vi "Thermal_Cycler_v0.3.vi"() -> ()   [LabVIEW 2023]
uses:
  <vilib>/Instr/_visa.llb/VISA Configure Serial Port (Instr).vi
panel:
  out "Flat Cycle Count":dbl
  out "Cold Count Readout":i32
  in  "Cold Count":i32
  in  "Cold Count Trigger":i32
  in  "Hot Count":i32
  in  "Hot Count Trigger":i32
  out "Full Temp Graph":dbl(graph)
  out "Cycle Temp Graph":dbl(graph)
  out "Current Cycle":i32
  out "Cycle Name":string
  out "Cooling":bool
  out "Heating":bool
  out "DONE":bool
  out "Soak High Adjusted":string
  out "Soak Low Adjusted":string
  in  "Multiplier":i32=60000
  out "Cycle Time in Minutes Adjusted":i32
  out "Temp Readout":dbl
  out "test read":string
  out "CYCLING":bool
  out "Was temp set correctly?":string
  in  "Comms delay":i32=1500
  in  "Number of Cycles to Complete":i32=2
  in  "Cycle Time in Minutes":i32=1
  in  "Soak Low":string="40"
  in  "Soak High":string="45"
  in  "baud rate":i32=19200
  out "ON/OFF":bool
  out "?":errorcluster
  in  "COM Port":refnum<visa-resource-name>="COM3"
  # "Debugging"
  # "Serial Port and Save Data Settings"
  # "Cycle and Temperature Settings"
  # "Readouts"
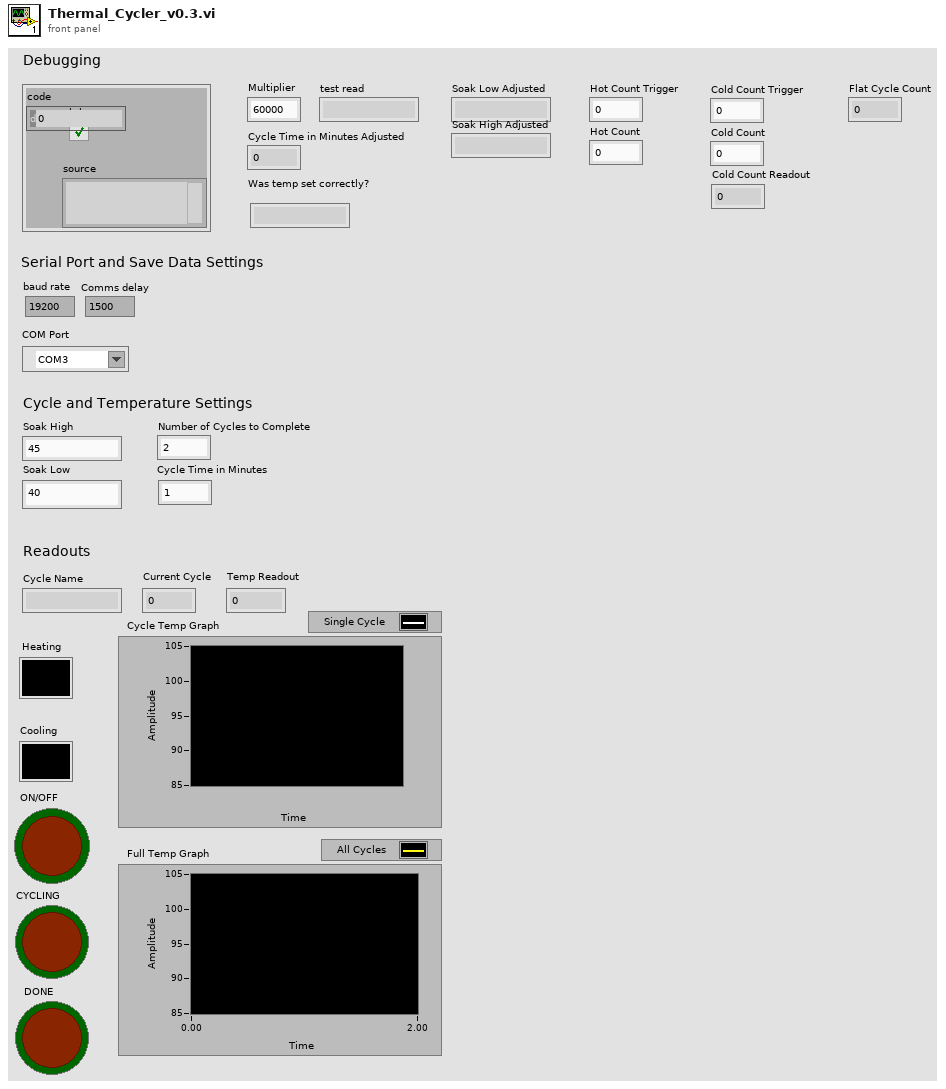
[diagram p1: front panel]
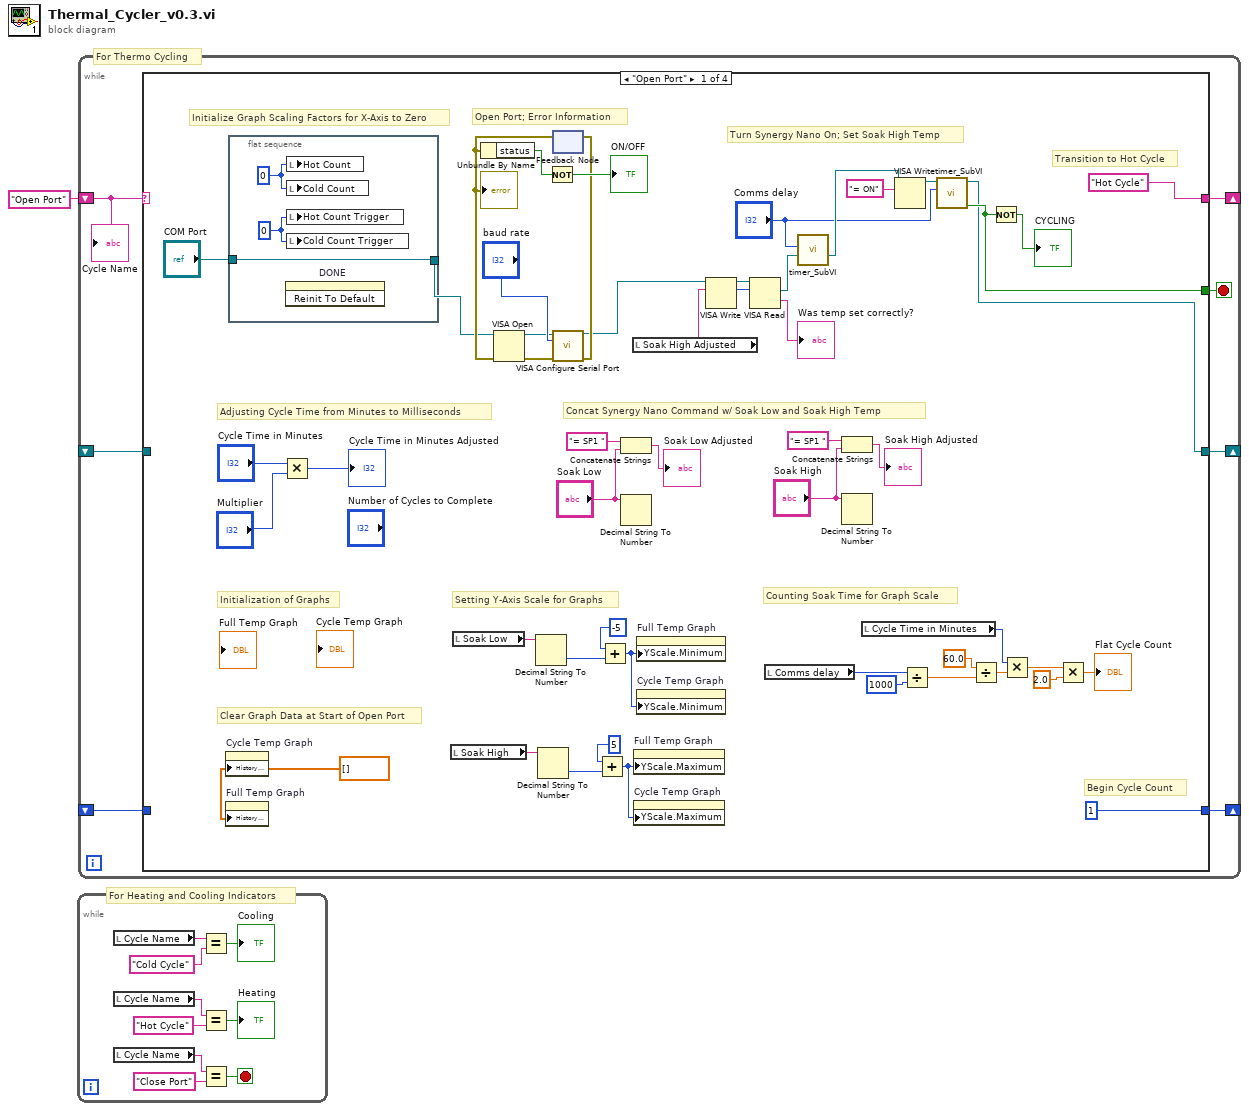
[diagram p0: block diagram]
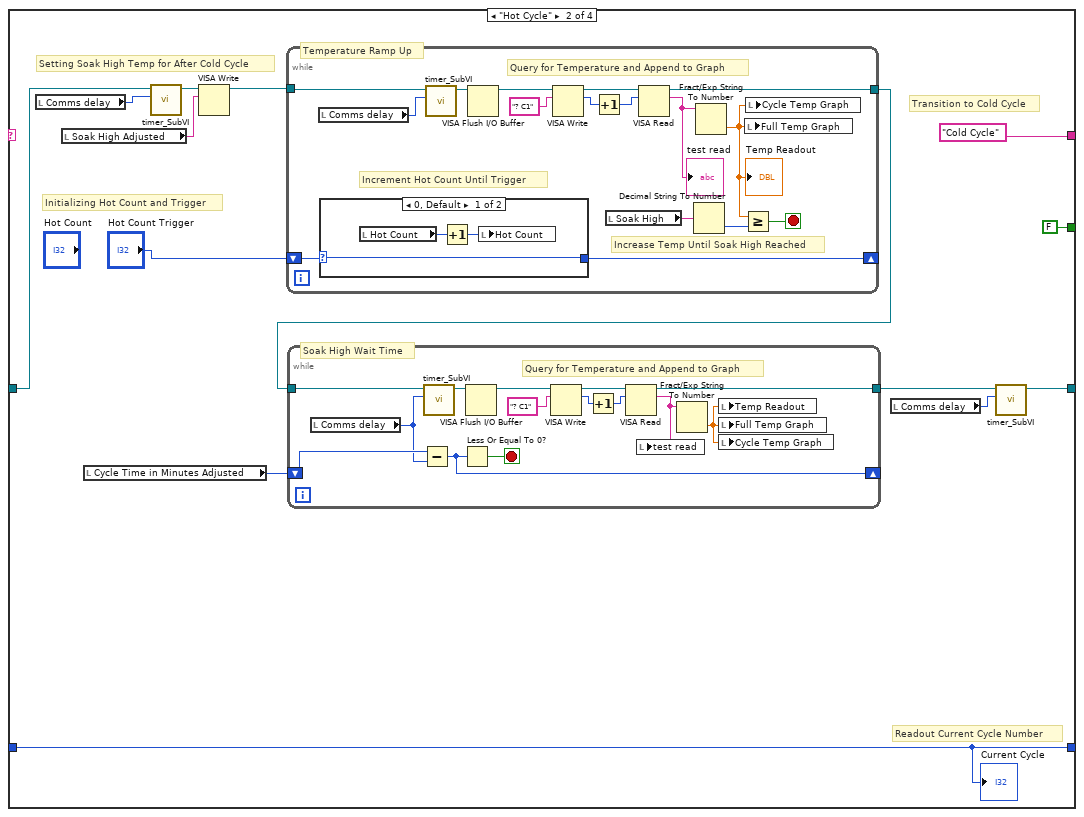
[diagram p2: hidden frame]
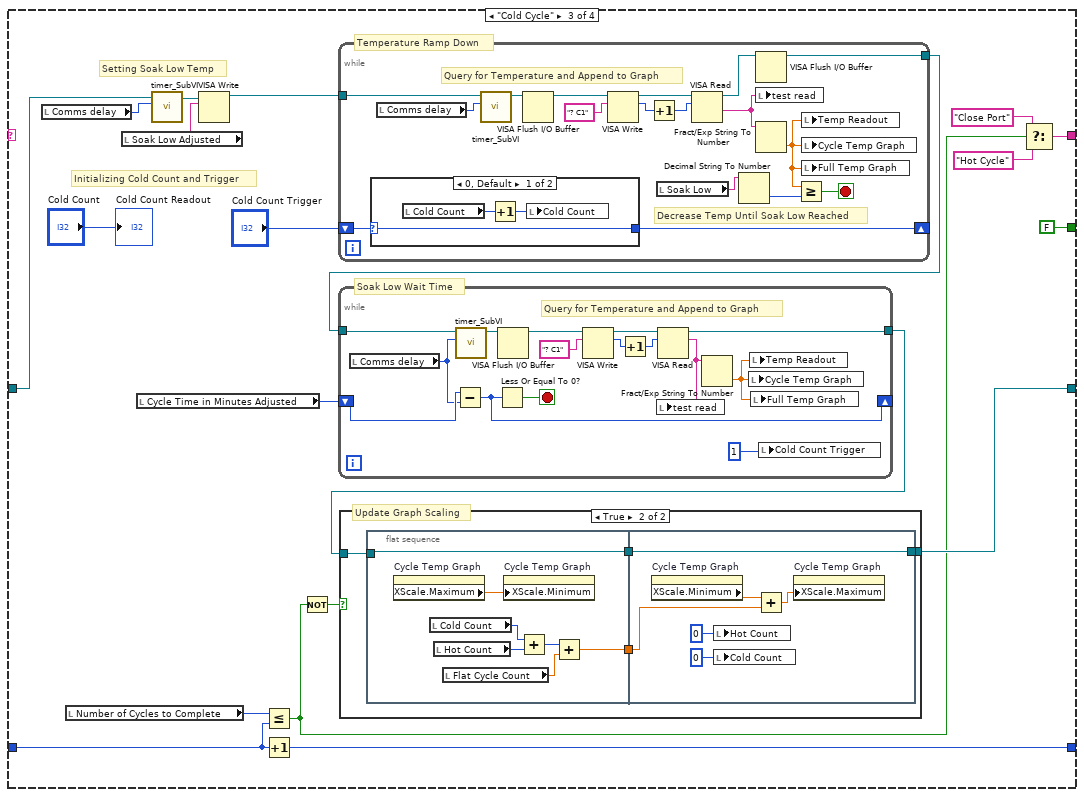
[diagram p4: hidden frame]
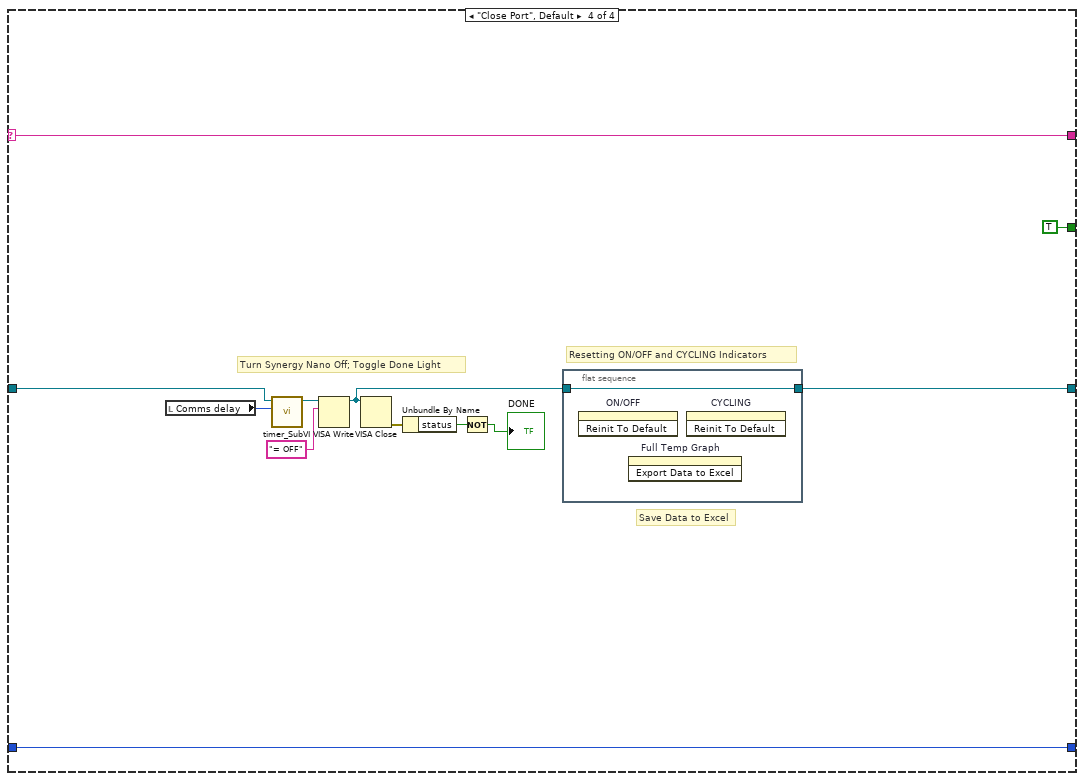
[diagram p7: hidden frame]
diagram:
  # "For Thermo Cycling"
  # "For Heating and Cooling Indicators"
  n1 = while {
    stop <- w2 stop-if-true
    n2 = local read "Cycle Name"() -> (w7:string)
    n3 = local read "Cycle Name"() -> (w10:string)
    n4 = local read "Cycle Name"() -> (w4:string)
    n5 = Equal?(x=w7, y="Cold Cycle") -> (x = y?=→"Cooling":bool)
    n6 = Equal?(x=w10, y="Hot Cycle") -> (x = y?=→"Heating":bool)
    n7 = Equal?(x=w4, y="Close Port") -> (x = y?=w2:bool)
  }
  n8 = while {
    shift-right: [w16] -> _
    shift-left: "Open Port" -> [w11]
    shift-right: [w15] -> _
    shift-left: _ -> [w14]
    shift-right: [w13] -> _
    shift-left: _ -> [w12]
    stop <- w17 stop-if-true
    n9 = case shown="\"Open Port\"" w11 {
      selector: w11 -> [_ _ _ w205]
      tunnel: [w46 FALSE FALSE TRUE] -> w17
      tunnel: ["Hot Cycle" "Cold Cycle" w128 w205] -> w16
      tunnel: [w44 w79 w122 w194] -> w15
      tunnel: w14 -> [_ w76 w134 w202]
      tunnel: [1 ("Numeric") w73 w126 w196] -> w13
      tunnel: w12 -> [_ w73 w127 w196]
      frame "Open Port" {
        w32 = dbl[] [] ("History Data")
        # "Transition to Hot Cycle"
        # "Begin Cycle Count"
        # "Turn Synergy Nano On; Set Soak High Temp"
        # "Open Port; Error Information"
        # "Initialize Graph Scaling Factors for X-Axis to Zero"
        # "Counting Soak Time for Graph Scale"
        # "Initialization of Graphs"
        # "Setting Y-Axis Scale for Graphs"
        # "Clear Graph Data at Start of Open Port"
        # "Adjusting Cycle Time from Minutes to Milliseconds"
        # "Concat Synergy Nano Command w/ Soak Low and Soak High Temp"
        n10 = property on="Cycle Temp Graph" class="WFChart (strict)"("History Data"=w32) -> ()  [unwired: 2 in, 2 out]
        n11 = property on="Full Temp Graph" class="WFChart (strict)"("History Data"=w32) -> ()  [unwired: 2 in, 2 out]
        n12 = flat-sequence {
          tunnel: "COM Port" -> [w71]
          tunnel: [w71] -> w30
          frame #0 {
            w69 = 0 ("Cold Count Trigger")
            w70 = 0 ("Cold Count")
            n13 = invoke on="DONE" class="Bool (strict)" method="Reinit To Default"() -> ()  [unwired: 3 in, 3 out]
            n14 = local write "Hot Count"(w70) -> ()
            n15 = local write "Cold Count"(w70) -> ()
            n16 = local write "Hot Count Trigger"(w69) -> ()
            n17 = local write "Cold Count Trigger"(w69) -> ()
          }
        }
        n18 = Multiply(x="Cycle Time in Minutes", y="Multiplier") -> (x*y=→"Cycle Time in Minutes Adjusted":i32)
        n19 = local read "Soak High"() -> (w34:string)
        n20 = local read "Soak Low"() -> (w33:string)
        n21 = Decimal String To Number(string=w33) -> (number=w41:i32)  [unwired: 2 in, 1 out]
        n22 = Decimal String To Number(string=w34) -> (number=w38:i32)  [unwired: 2 in, 1 out]
        n23 = feedback #1() -> (w60:errorcluster)  [unwired: 1 in]
        "?" <- w60
        n24 = Unbundle By Name(w60) -> ("status"=w65:bool)
        n25 = VISA Open(error in (no error)=w60, VISA resource name=w30) -> (VISA resource name=w66:refnum<visa-resource-name>, error out=w68:errorcluster)  [unwired: 3 in]
        n26 = Not(x=w65) -> (.not. x?=→"ON/OFF":bool)
        n27 = call-poly "VISA Configure Serial Port"("VISA resource name"=w66, "baud rate (9600)"="baud rate", "error in (no error)"=w68) -> ("VISA resource name out"=w47:refnum<visa-resource-name>, "error out"=w61:errorcluster)  [unwired: 11 in]
        n28 = feedback-in #1(w61) -> ()
        n29 = Add(x=5, y=w38) -> (x+y=w35:i32)
        n30 = Add(x=-5, y=w41) -> (x+y=w39:i32)
        n31 = Concatenate Strings("= SP1 ", "Soak Low") -> (→"Soak Low Adjusted":string)
        n32 = Decimal String To Number(string="Soak Low") -> ()  [unwired: 2 in, 2 out]
        n33 = local read "Soak High Adjusted"() -> (w20:string)
        n34 = property on="Full Temp Graph" class="WFChart (strict)"("YScale.Maximum"=w35) -> ()  [unwired: 2 in, 2 out]
        n35 = property on="Cycle Temp Graph" class="WFChart (strict)"("YScale.Maximum"=w35) -> ()  [unwired: 2 in, 2 out]
        n36 = property on="Full Temp Graph" class="WFChart (strict)"("YScale.Minimum"=w39) -> ()  [unwired: 2 in, 2 out]
        n37 = property on="Cycle Temp Graph" class="WFChart (strict)"("YScale.Minimum"=w39) -> ()  [unwired: 2 in, 2 out]
        n38 = VISA Write(VISA resource name=w47, write buffer=w20) -> (VISA resource name out=w48:refnum<visa-resource-name>, return count=w49:u32)  [unwired: 1 in, 1 out]
        n39 = VISA Read(VISA resource name=w48, byte count=w49) -> (VISA resource name out=w59:refnum<visa-resource-name>, read buffer=→"Was temp set correctly?":string)  [unwired: 1 in, 2 out]
        n40 = local read "Comms delay"() -> (w28:i32)
        n41 = call "timer_SubVI.vi"("Comms Delay In"="Comms delay", "VISA  in"=w59) -> ("VISA out"=w56:refnum<visa-resource-name>)  [unwired: 7 in, 2 out]
        n42 = Concatenate Strings("= SP1 ", "Soak High") -> (→"Soak High Adjusted":string)
        n43 = Decimal String To Number(string="Soak High") -> ()  [unwired: 2 in, 2 out]
        n44 = local read "Cycle Time in Minutes"() -> (w29:i32)
        n45 = VISA Write(VISA resource name=w56, write buffer="= ON") -> (VISA resource name out=w55:refnum<visa-resource-name>)  [unwired: 1 in, 2 out]
        n46 = Divide(x=w28, y=1000) -> (x/y=w25:dbl)
        n47 = call "timer_SubVI.vi"("Comms Delay In"="Comms delay", "VISA  in"=w55) -> ("bool out"=w46:bool, "VISA out"=w44:refnum<visa-resource-name>)  [unwired: 7 in, 1 out]
        n48 = Divide(x=60.0 ("y"), y=w25) -> (x/y=w24:dbl)
        n49 = Not(x=w46) -> (.not. x?=→"CYCLING":bool)
        n50 = Multiply(x=w29, y=w24) -> (x*y=w23:dbl)
        n51 = Multiply(x=w23, y=2.0) -> (x*y=→"Flat Cycle Count":dbl)
      }
      frame "Hot Cycle" {
        # "Transition to Cold Cycle"
        # "Readout Current Cycle Number"
        # "Soak High Wait Time"
        # "Initializing Hot Count and Trigger"
        # "Setting Soak High Temp for After Cold Cycle"
        # "Temperature Ramp Up"
        n52 = local read "Comms delay"() -> (w74:i32)
        n53 = local read "Soak High Adjusted"() -> (w83:string)
        n54 = local read "Cycle Time in Minutes Adjusted"() -> (w81:i32)
        n55 = call "timer_SubVI.vi"("Comms Delay In"=w74, "VISA  in"=w76) -> ("VISA out"=w75:refnum<visa-resource-name>)  [unwired: 7 in, 2 out]
        n56 = VISA Write(VISA resource name=w75, write buffer=w83) -> (VISA resource name out=w84:refnum<visa-resource-name>)  [unwired: 1 in, 2 out]
        n57 = while {
          tunnel: [w109] -> w82
          tunnel: w84 -> [w108]
          shift-right: [w100] -> _
          shift-left: "Hot Count Trigger" -> [w101]
          stop <- w112 stop-if-true
          # "Increase Temp Until Soak High Reached"
          # "Query for Temperature and Append to Graph"
          # "Increment Hot Count Until Trigger"
          n58 = local read "Comms delay"() -> (w107:i32)
          n59 = case shown="0, Default" w101 {
            selector: w101 -> [w116 w119]
            tunnel: [w116 w119] -> w100
            frame 0, Default {
              n60 = local read "Hot Count"() -> (w118:i32)
              n61 = Increment(x=w118) -> (x+1=w117:i32)
              n62 = local write "Hot Count"(w117) -> ()
            }
            frame 1 {
            }
          }
          n63 = call "timer_SubVI.vi"("Comms Delay In"=w107, "VISA  in"=w108) -> ("VISA out"=w104:refnum<visa-resource-name>)  [unwired: 7 in, 2 out]
          n64 = VISA Flush I/O Buffer(VISA resource name=w104) -> (VISA resource name out=w103:refnum<visa-resource-name>)  [unwired: 2 in, 1 out]
          n65 = VISA Write(VISA resource name=w103, write buffer="? C1") -> (VISA resource name out=w115:refnum<visa-resource-name>, return count=w111:u32)  [unwired: 1 in, 1 out]
          n66 = Increment(x=w111) -> (x+1=w110:u32)
          n67 = local read "Soak High"() -> (w106:string)
          n68 = VISA Read(VISA resource name=w115, byte count=w110) -> (VISA resource name out=w109:refnum<visa-resource-name>, read buffer=w114:string)  [unwired: 1 in, 2 out]
          "test read" <- w114
          n69 = Decimal String To Number(string=w106) -> (number=w105:i32)  [unwired: 2 in, 1 out]
          n70 = Fract/Exp String To Number(string=w114) -> (number=w102:dbl)  [unwired: 3 in, 1 out]
          "Temp Readout" <- w102
          n71 = Greater Or Equal?(x=w102, y=w105) -> (x >= y?=w112:bool)
          n72 = local write "Full Temp Graph"(w102) -> ()
          n73 = local write "Cycle Temp Graph"(w102) -> ()
        }
        n74 = while {
          tunnel: w82 -> [w88]
          tunnel: [w96] -> w80
          shift-right: [w94] -> _
          shift-left: w81 -> [w95]
          stop <- w99 stop-if-true
          # "Query for Temperature and Append to Graph"
          n75 = local read "Comms delay"() -> (w89:i32)
          n76 = Subtract(x=w95, y=w89) -> (x-y=w94:i32)
          n77 = call "timer_SubVI.vi"("Comms Delay In"=w89, "VISA  in"=w88) -> ("VISA out"=w87:refnum<visa-resource-name>)  [unwired: 7 in, 2 out]
          n78 = Less Or Equal To 0?(x=w94) -> (x <= 0?=w99:bool)
          n79 = VISA Flush I/O Buffer(VISA resource name=w87) -> (VISA resource name out=w86:refnum<visa-resource-name>)  [unwired: 2 in, 1 out]
          n80 = VISA Write(VISA resource name=w86, write buffer="? C1") -> (VISA resource name out=w98:refnum<visa-resource-name>, return count=w91:u32)  [unwired: 1 in, 1 out]
          n81 = Increment(x=w91) -> (x+1=w90:u32)
          n82 = VISA Read(VISA resource name=w98, byte count=w90) -> (VISA resource name out=w96:refnum<visa-resource-name>, read buffer=w92:string)  [unwired: 1 in, 2 out]
          n83 = local write "test read"(w92) -> ()
          n84 = Fract/Exp String To Number(string=w92) -> (number=w93:dbl)  [unwired: 3 in, 1 out]
          n85 = local write "Temp Readout"(w93) -> ()
          n86 = local write "Full Temp Graph"(w93) -> ()
          n87 = local write "Cycle Temp Graph"(w93) -> ()
        }
        n88 = local read "Comms delay"() -> (w78:i32)
        n89 = call "timer_SubVI.vi"("Comms Delay In"=w78, "VISA  in"=w80) -> ("VISA out"=w79:refnum<visa-resource-name>)  [unwired: 7 in, 2 out]
        "Current Cycle" <- w73
      }
      frame "Cold Cycle" {
        # "Update Graph Scaling"
        # "Initializing Cold Count and Trigger"
        # "Setting Soak Low Temp"
        # "Soak Low Wait Time"
        # "Temperature Ramp Down"
        n90 = local read "Comms delay"() -> (w135:i32)
        n91 = local read "Number of Cycles to Complete"() -> (w131:i32)
        n92 = local read "Soak Low Adjusted"() -> (w137:string)
        n93 = local read "Cycle Time in Minutes Adjusted"() -> (w136:i32)
        n94 = call "timer_SubVI.vi"("Comms Delay In"=w135, "VISA  in"=w134) -> ("VISA out"=w133:refnum<visa-resource-name>)  [unwired: 7 in, 2 out]
        n95 = VISA Write(VISA resource name=w133, write buffer=w137) -> (VISA resource name out=w132:refnum<visa-resource-name>)  [unwired: 1 in, 2 out]
        n96 = Less Or Equal?(x=w131, y=w127) -> (x <= y?=w120:bool)
        n97 = Increment(x=w127) -> (x+1=w126:i32)
        n98 = Not(x=w120) -> (.not. x?=w123:bool)
        n99 = while {
          tunnel: [w185] -> w138
          tunnel: w132 -> [w183]
          shift-right: [w175] -> _
          shift-left: "Cold Count Trigger" -> [w176]
          stop <- w188 stop-if-true
          # "Decrease Temp Until Soak Low Reached"
          # "Query for Temperature and Append to Graph"
          n100 = case shown="0, Default" w176 {
            selector: w176 -> [w190 w193]
            tunnel: [w190 w193] -> w175
            frame 0, Default {
              n101 = local read "Cold Count"() -> (w192:i32)
              n102 = Increment(x=w192) -> (x+1=w191:i32)
              n103 = local write "Cold Count"(w191) -> ()
            }
            frame 1 {
            }
          }
          n104 = local read "Comms delay"() -> (w182:i32)
          n105 = call "timer_SubVI.vi"("Comms Delay In"=w182, "VISA  in"=w183) -> ("VISA out"=w178:refnum<visa-resource-name>)  [unwired: 7 in, 2 out]
          n106 = VISA Flush I/O Buffer(VISA resource name=w178) -> (VISA resource name out=w177:refnum<visa-resource-name>)  [unwired: 2 in, 1 out]
          n107 = VISA Write(VISA resource name=w177, write buffer="? C1") -> (VISA resource name out=w179:refnum<visa-resource-name>, return count=w187:u32)  [unwired: 1 in, 1 out]
          n108 = Increment(x=w187) -> (x+1=w186:u32)
          n109 = local read "Soak Low"() -> (w180:string)
          n110 = VISA Read(VISA resource name=w179, byte count=w186) -> (VISA resource name out=w184:refnum<visa-resource-name>, read buffer=w181:string)  [unwired: 1 in, 2 out]
          n111 = Decimal String To Number(string=w180) -> (number=w173:i32)  [unwired: 2 in, 1 out]
          n112 = VISA Flush I/O Buffer(VISA resource name=w184) -> (VISA resource name out=w185:refnum<visa-resource-name>)  [unwired: 2 in, 1 out]
          n113 = local write "test read"(w181) -> ()
          n114 = Fract/Exp String To Number(string=w181) -> (number=w174:dbl)  [unwired: 3 in, 1 out]
          n115 = Greater Or Equal?(x=w174, y=w173) -> (x >= y?=w188:bool)
          n116 = local write "Temp Readout"(w174) -> ()
          n117 = local write "Cycle Temp Graph"(w174) -> ()
          n118 = local write "Full Temp Graph"(w174) -> ()
        }
        n119 = while {
          tunnel: w138 -> [w169]
          tunnel: [w168] -> w121
          shift-right: [w166] -> _
          shift-left: w136 -> [w167]
          stop <- w172 stop-if-true
          # "Query for Temperature and Append to Graph"
          n120 = local read "Comms delay"() -> (w161:i32)
          n121 = Subtract(x=w167, y=w161) -> (x-y=w166:i32)
          n122 = call "timer_SubVI.vi"("Comms Delay In"=w161, "VISA  in"=w169) -> ("VISA out"=w160:refnum<visa-resource-name>)  [unwired: 7 in, 2 out]
          n123 = Less Or Equal To 0?(x=w166) -> (x <= 0?=w172:bool)
          n124 = VISA Flush I/O Buffer(VISA resource name=w160) -> (VISA resource name out=w159:refnum<visa-resource-name>)  [unwired: 2 in, 1 out]
          n125 = VISA Write(VISA resource name=w159, write buffer="? C1") -> (VISA resource name out=w171:refnum<visa-resource-name>, return count=w163:u32)  [unwired: 1 in, 1 out]
          n126 = Increment(x=w163) -> (x+1=w162:u32)
          n127 = VISA Read(VISA resource name=w171, byte count=w162) -> (VISA resource name out=w168:refnum<visa-resource-name>, read buffer=w164:string)  [unwired: 1 in, 2 out]
          n128 = local write "test read"(w164) -> ()
          n129 = Fract/Exp String To Number(string=w164) -> (number=w165:dbl)  [unwired: 3 in, 1 out]
          n130 = local write "Cycle Temp Graph"(w165) -> ()
          n131 = local write "Temp Readout"(w165) -> ()
          n132 = local write "Full Temp Graph"(w165) -> ()
          n133 = local write "Cold Count Trigger"(1 ("Numeric")) -> ()
        }
        n134 = case shown="True" w123 {
          tunnel: [w140 w144] -> w122
          tunnel: w121 -> [w140 w143]
          frame False {
          }
          frame True {
            n135 = flat-sequence {
              tunnel: w143 -> [w147]
              tunnel: [w147] -> w142
              tunnel: [w146] -> w141
              tunnel: [w157] -> w144
              tunnel: w142 -> [w157]
              tunnel: w141 -> [w153]
              frame #0 {
                n136 = property on="Cycle Temp Graph" class="WFChart (strict)"() -> ("XScale.Maximum"=w145:dbl)  [unwired: 2 in, 2 out]
                n137 = local read "Cold Count"() -> (w151:i32)
                n138 = local read "Hot Count"() -> (w149:i32)
                n139 = local read "Flat Cycle Count"() -> (w148:dbl)
                n140 = property on="Cycle Temp Graph" class="WFChart (strict)"("XScale.Minimum"=w145) -> ()  [unwired: 2 in, 2 out]
                n141 = Add(x=w151, y=w149) -> (x+y=w150:i32)
                n142 = Add(x=w150, y=w148) -> (x+y=w146:dbl)
              }
              frame #1 {
                n143 = property on="Cycle Temp Graph" class="WFChart (strict)"() -> ("XScale.Minimum"=w152:dbl)  [unwired: 2 in, 2 out]
                n144 = local write "Hot Count"(0 ("Cold Count")) -> ()
                n145 = local write "Cold Count"(0 ("Cold Count")) -> ()
                n146 = Add(x=w152, y=w153) -> (x+y=w154:dbl)
                n147 = property on="Cycle Temp Graph" class="WFChart (strict)"("XScale.Maximum"=w154) -> ()  [unwired: 2 in, 2 out]
              }
            }
          }
        }
        n148 = Select(t="Close Port", s=w120, f="Hot Cycle") -> (s? t:f=w128:string)
        "Cold Count Readout" <- "Cold Count"
      }
      frame "Close Port", Default {
        # "Save Data to Excel"
        # "Resetting ON/OFF and CYCLING Indicators"
        # "Turn Synergy Nano Off; Toggle Done Light"
        n149 = local read "Comms delay"() -> (w203:i32)
        n150 = call "timer_SubVI.vi"("Comms Delay In"=w203, "VISA  in"=w202) -> ("VISA out"=w198:refnum<visa-resource-name>)  [unwired: 7 in, 2 out]
        n151 = VISA Write(VISA resource name=w198, write buffer="= OFF") -> (VISA resource name out=w195:refnum<visa-resource-name>)  [unwired: 1 in, 2 out]
        n152 = VISA Close(VISA resource name=w195) -> (error out=w197:errorcluster)  [unwired: 1 in]
        n153 = Unbundle By Name(w197) -> ("status"=w199:bool)
        n154 = Not(x=w199) -> (.not. x?=→"DONE":bool)
        n155 = flat-sequence {
          tunnel: w195 -> [w206]
          tunnel: [w206] -> w194
          frame #0 {
            n156 = invoke on="ON/OFF" class="Bool (strict)" method="Reinit To Default"() -> ()  [unwired: 3 in, 3 out]
            n157 = invoke on="Full Temp Graph" class="WFChart (strict)" method="Export Data to Excel"() -> ()  [unwired: 3 in, 3 out]
            n158 = invoke on="CYCLING" class="Bool (strict)" method="Reinit To Default"() -> ()  [unwired: 3 in, 3 out]
          }
        }
      }
    }
    "Cycle Name" <- w11
  }
